vi "Field Sweep.vi"() -> ()   [LabVIEW 8.6]
uses:
  <vilib>/Platform/TimedLoop/XDataNode/XDataNode.xnode
  <vilib>/Platform/TimedLoop/XDataNode/nitl_modes.ctl
  <vilib>/Platform/TimedLoop/XDataNode/XDNodeRunTimeDep.lvlib
  <vilib>/Platform/TimedLoop/XDataNode/wakeup.ctl
  <vilib>/Platform/TimedLoop/XDataNode/timing_clust.ctl
  <vilib>/Platform/TimedLoop/XDataNode/loadlvalarms.vi
panel:
  out "Finished 2":bool
  in  "Step Size":dbl
  out "set 3":dbl
  out "Field":dbl
  out "Finished":bool
  in  "Go":bool
  in  "Stop":dbl
  in  "Start":dbl
  in  "Sweep Rate (sec/step)":dbl
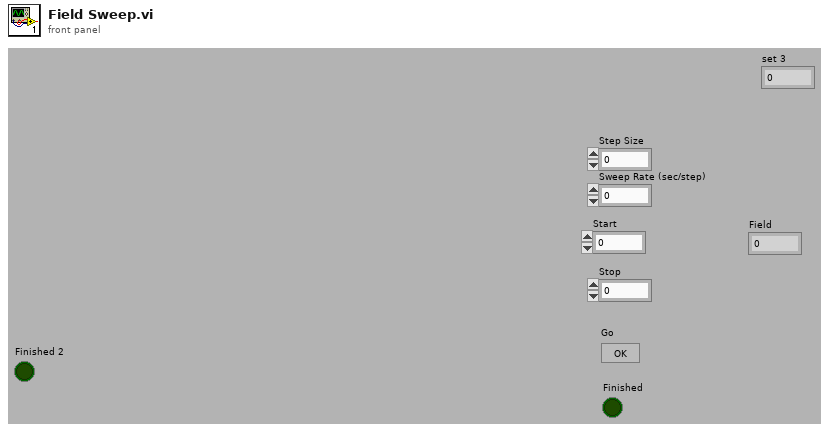
[diagram p1: front panel]
types:
  T1 = typedef "XDNodeRunTimeDep.lvlib/timing_clust.ctl" = cluster{"Expected End [f-1]":u64, "Actual End [f-1]":u64, "Finished Late? [f-1]":bool, "Expected End [i-1]":u64, "Actual End [i-1]":u64, "Finished Late? [i-1]":bool, "Expected Start [i]":u64, "Actual Start [i]":u64, "Expected Start [f]":u64, "Actual Start [f]":u64, "Source Name":string, "Structure Name":string, "Period":i64, "Deadline":i64, "Offset":i64, "Start":i64, "Priority":i32, "Timeout":i32, "Mode":T2, "Wakeup Reason":T3, "Error":errorcluster, "Source Type":string, "Secondary Source Type":string, "Global End Time":u64, "Global Start Time":u64, "Frame Duration":u64, "Iteration Duration":u64, "Assigned CPU":i32, "I/O Scan Engine Mode":u32}
  T2 = typedef "XDNodeRunTimeDep.lvlib/nitl_modes.ctl" = enum32{"No Change", "Process missed periods, maintain original phase", "Discard missed periods, maintain original phase", "Process missed periods, ignore original phase", "Discard missed periods, ignore original phase"}
  T3 = typedef "XDNodeRunTimeDep.lvlib/wakeup.ctl" = enum32{"Normal", "Aborted", "Asynchronous wakeup", "Timing source error", "Timed loop error", "Timeout"}
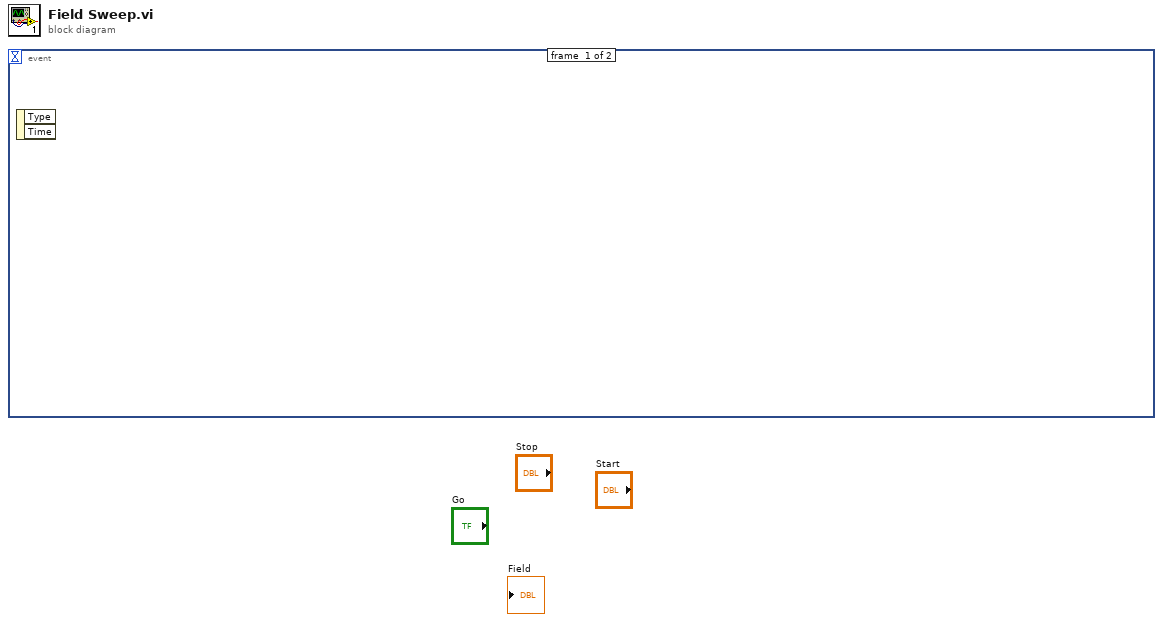
[diagram p0: block diagram]
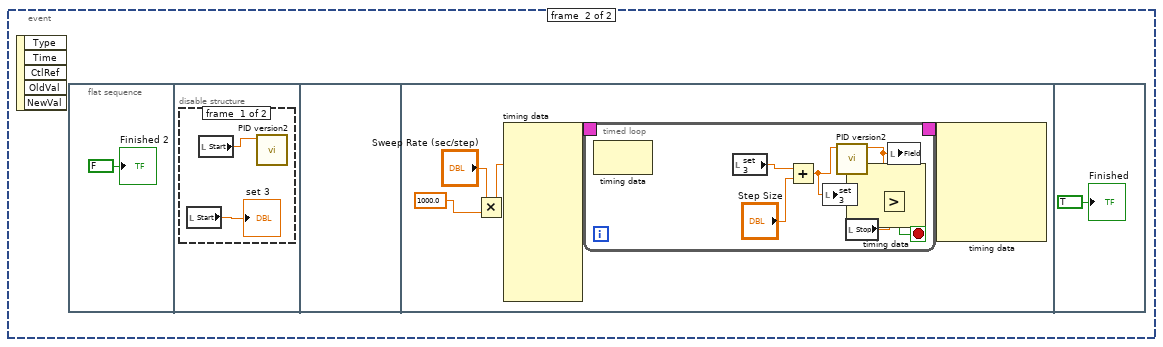
[diagram p2: hidden frame]
diagram:
  n1 = event shown="[1] \"Go\": Value Change" {
    selector: _ -> [_ _]
    dyn-events: _ -> [_ _]
    timeout: _ -> [_ _]
    event #0 {
      n2 = event-data() -> ()  [unwired: 1 in, 2 out]
    }
    event #1 {
      n3 = event-data() -> ()  [unwired: 1 in, 5 out]
      n4 = flat-sequence {
        frame #0 {
          "Finished 2" <- FALSE ("Finished")
        }
        frame #1 {
          n5 = disable-structure shown="Enabled" {
            frame #0 {
              n6 = local read "Start"() -> (→"set 3":dbl)
              n7 = local read "Start"() -> (w3:dbl)
              n8 = call "PID version2.vi"("Field Desired (T)"=w3) -> ()  [unwired: 10 in, 1 out]
            }
            frame #1 {
            }
          }
        }
        frame #2 {
        }
        frame #3 {
          n9 = Multiply(x="Sweep Rate (sec/step)", y=1000.0) -> (x*y=w4:dbl)
          n10 = node-c288(w4) -> (w8:T1)  [unwired: 9 in]
          n11 = timed-loop {
            timing: w8 -> [_]
            timing-out: [_] -> w7
            stop <- w11 stop-if-true
            n12 = node-c288() -> ()  [unwired: 1 in, 1 out]
            n13 = local read "set 3"() -> (w14:dbl)
            n14 = Add(x=w14, y="Step Size") -> (x+y=w12:dbl)
            n15 = local write "set 3"(w12) -> ()
            n16 = call "PID version2.vi"("Field Desired (T)"=w12) -> ("Tesla"=w9:dbl)  [unwired: 10 in]
            n17 = local read "Stop"() -> (w10:dbl)
            n18 = node-c288() -> ()  [unwired: 3 in, 1 out]
            n19 = Greater?(x=w9, y=w10) -> (0:w11:bool)
            n20 = local write "Field"(w9) -> ()
          }
          n21 = node-c288(w7) -> ()  [unwired: 6 out]
        }
        frame #4 {
          "Finished" <- TRUE ("Finished")
        }
      }
    }
  }
